vi "IT-Test.vi"() -> ()   [LabVIEW 2014]
uses:
  <vilib>/httpClient/POSTBuffer.vi
  <vilib>/httpClient/LabVIEWHTTPClient.lvlib
panel:
  out "headers":string="HTTP/1.1 200 OK\r\nCache-Control: no-cache\r\nPragma: no-cache\r\nContent-Length: 27\r\nContent-Type: application/json; charset=utf-8\r\nExpires: -1\r\nServer: Microsoft-IIS/7.5\r\nX-AspNet-Version: 4.0.30319\r\nX-Powered-By: ASP.NET\r\nDate: Fri, 10 Nov 2017 02:26:55 GMT\r\n\r\n"
  out "error out":errorcluster
  in  "error in (no error)":errorcluster
  in  "CARNO":string="01"
  in  "BARCODE2":string="%7123450"
  in  "BARCODE2M":string="TH-32C400W"
  in  "PRODCODE":string="1213"
  out "Message":string="save ok"
  out "body":string="{\"RC\":\"save ok\",\"TOTALY\":2}"
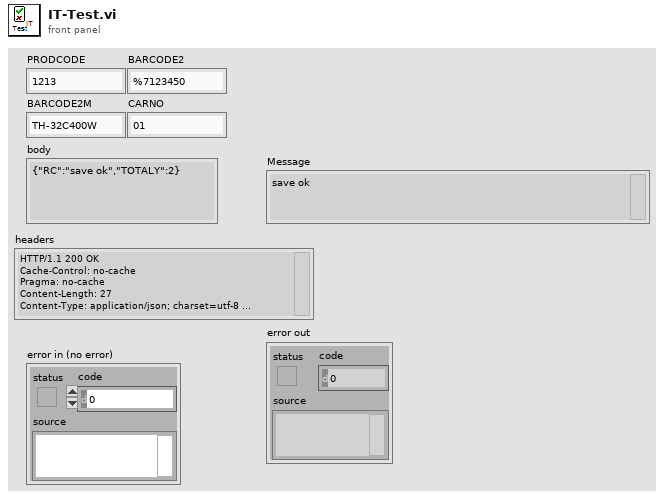
[diagram p1: front panel]
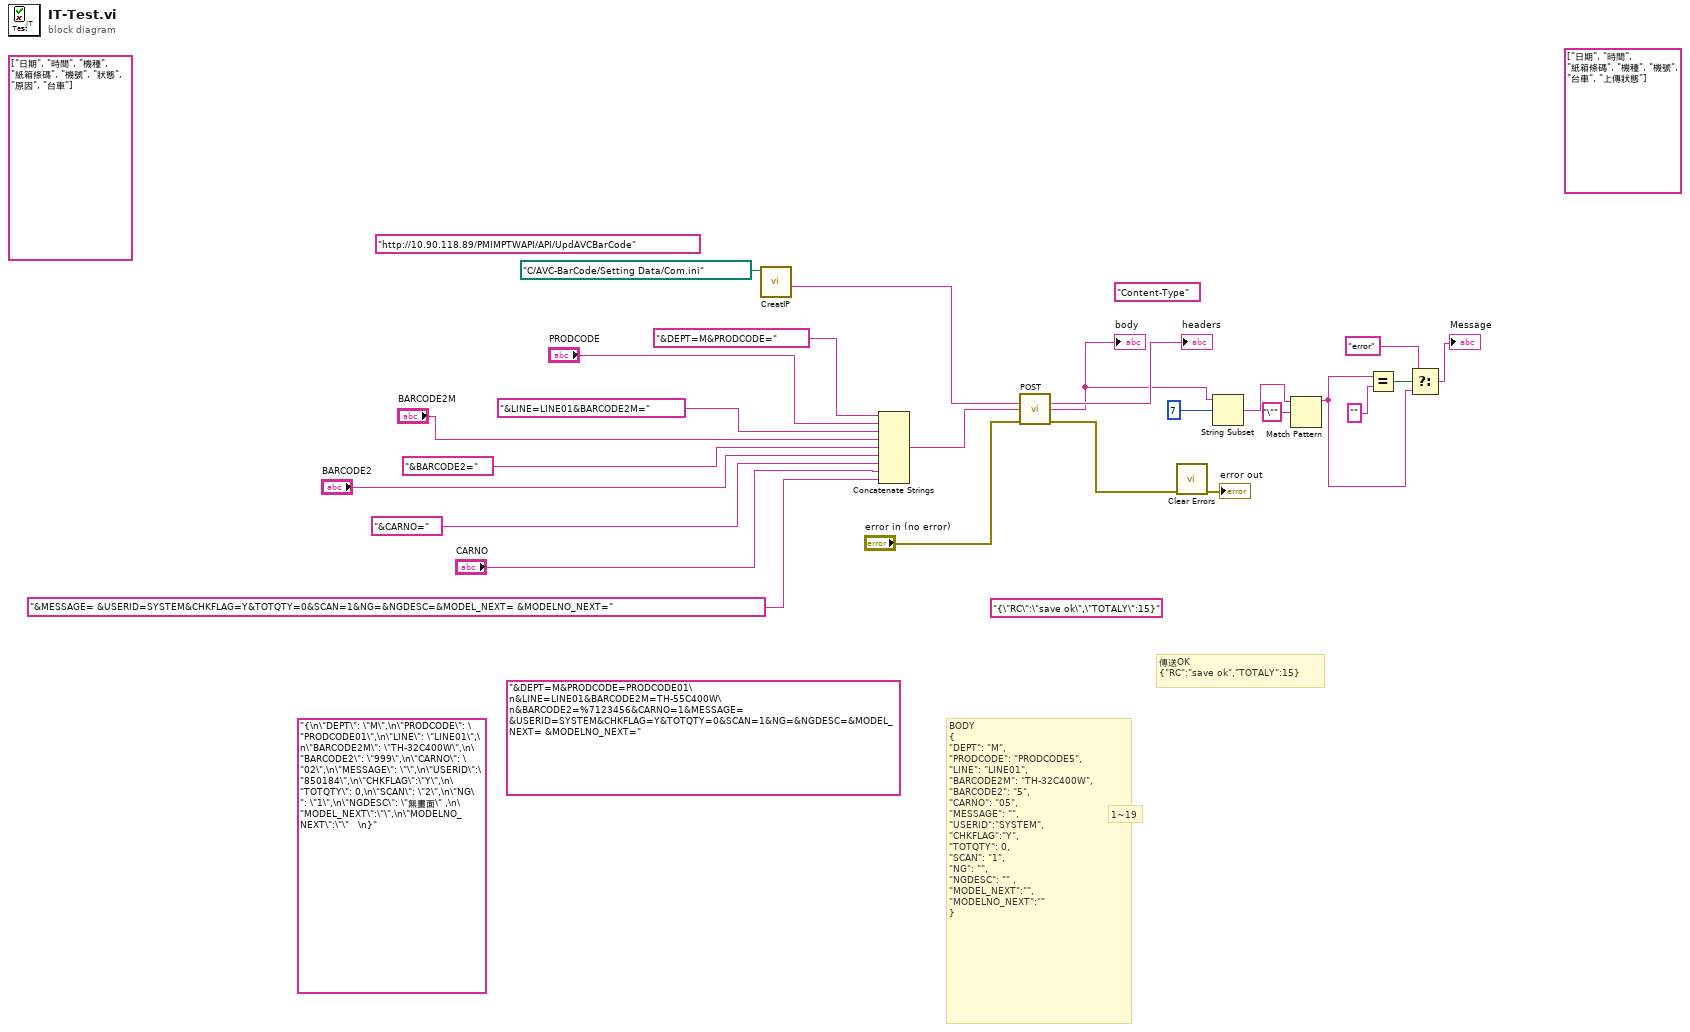
[diagram p0: block diagram]
diagram:
  (unwired) string[] ["日期", "時間", "紙箱條碼", "機種", "機號", "台車", "上傳狀態"]
  (unwired) string[] ["日期", "時間", "機種", "紙箱條碼", "機號", "狀態", "原因", "台車"]
  (unwired) "{\"RC\":\"save ok\",\"TOTALY\":15}"
  (unwired) "&DEPT=M&PRODCODE=PRODCODE01\n&LINE=LINE01&BARCODE2M=TH-55C400W\n&BARCODE2=%7123456&CARNO=1&MESSAGE= &USERID=SYSTEM&CHKFLAG=Y&TOTQTY=0&SCAN=1&NG=&NGDESC=&MODEL_NEXT= &MODELNO_NEXT="
  (unwired) "{\n\"DEPT\": \"M\",\n\"PRODCODE\": \"PRODCODE01\",\n\"LINE\": \"LINE01\",\n\"BARCODE2M\": \"TH-32C400W\",\n\"BARCODE2\": \"999\",\n\"CARNO\": \"02\",\n\"MESSAGE\": \"\",\n\"USERID\":\"850184\",\n\"CHKFLAG\":\"Y\",\n\"TOTQTY\": 0,\n\"SCAN\": \"2\",\n\"NG\": \"1\",\n\"NGDESC\": \"無畫面\" ,\n\"MODEL_NEXT\":\"\",\n\"MODELNO_NEXT\":\"\"   \n}" ("buffer")
  (unwired) "Content-Type" ("body")
  (unwired) "http://10.90.118.89/PMIMPTWAPI/API/UpdAVCBarCode" ("url")
  # "傳送OK\n{\"RC\":\"save ok\",\"TOTALY\":15}"
  # "BODY\n{\n\"DEPT\": \"M\",\n\"PRODCODE\": \"PRODCODE5\",\n\"LINE\": \"LINE01\",\n\"BARCODE2M\": \"TH-32C400W\",\n\"BARCODE2\": \"5\",\n\"CARNO\": \"05\",\n\"MESSAGE\": \"\",\n\"USERID\":\"SYSTEM\",\n\"CHKFLAG\":\"Y\",\n\"TOTQTY\": 0,\n\"SCAN\": \"1\",\n\"NG\": \"\",\n\"NGDESC\": \"\" ,\n\"MODEL_NEXT\":\"\",\n\"MODELNO_NEXT\":\"\" \n}"
  # "1~19"
  n1 = call "CreatIP.vi"("file Path"=path "C:/AVC-BarCode/Setting Data/Com.ini") -> ("IT IP"=w16:string)  [unwired: 8 in, 2 out]
  n2 = Concatenate Strings("&DEPT=M&PRODCODE=" ("string"), "PRODCODE", "&LINE=LINE01&BARCODE2M=" ("string"), "BARCODE2M", "&BARCODE2=" ("string"), "BARCODE2", "&CARNO=" ("string"), "CARNO", "&MESSAGE= &USERID=SYSTEM&CHKFLAG=Y&TOTQTY=0&SCAN=1&NG=&NGDESC=&MODEL_NEXT= &MODELNO_NEXT=") -> (w20:string)
  n3 = call-poly <vilib>:"POST.vi"("url"=w16, "buffer"=w20, "error in (no error)"="error in (no error)") -> ("headers"=→"headers":string, "body"=w12:string, "error out"=w18:errorcluster)  [unwired: 9 in, 1 out]
  "body" <- w12
  n4 = call <vilib>:"Clear Errors.vi"("error in (no error)"=w18) -> ("error out"=→"error out":errorcluster)  [unwired: 5 in, 1 out]
  n5 = String Subset(string=w12, offset (0)=7) -> (substring=w10:string)  [unwired: 1 in]
  n6 = Match Pattern(string=w10, regular expression="\"") -> (before substring=w7:string)  [unwired: 1 in, 3 out]
  n7 = Equal?(x=w7, y="") -> (x = y?=w8:bool)
  n8 = Select(t="error", s=w8, f=w7) -> (s? t:f=→"Message":string)
